vi "Extract K-Clock Phase Using Hilbert.vi"(7 "window":T1 items=["Rectangle"=0, "Hanning"=1, "Hamming"=2, "Blackman-Harris"=3, "Exact Blackman"=4, "Blackman"=5, "Flat Top"=6, "4 Term B-Harris "=7, "7 Term B-Harris"=8, "Low Sidelobe"=9, "Blackman Nuttall"=11, "Triangle"=30, "Bartlett-Hanning"=31, "Bohman"=32, "Parzen"=33, "Welch"=34, "Kaiser"=60, "Dolph-Chebyshev"=61, "Gaussian"=62], 11 "Input Data":dbl[](array[numeric]) format="%0.2f") -> (3 "Hilbert Unwrapped Phase":dbl[](array[numeric]))   [LabVIEW 2012]
uses:
  <vilib>/Analysis/4window.llb/windowTd.ctl
  <vilib>/Analysis/baseanly.llb/Mean (DBL).vi
  <vilib>/Analysis/0measdsp.llb/Scaled Time Domain Window (DBL).vi
  <vilib>/Analysis/NI_AALPro.lvlib
  <vilib>/Analysis/NI_AALBase.lvlib
panel:
  out "Hilbert Phase":dbl[](graph)
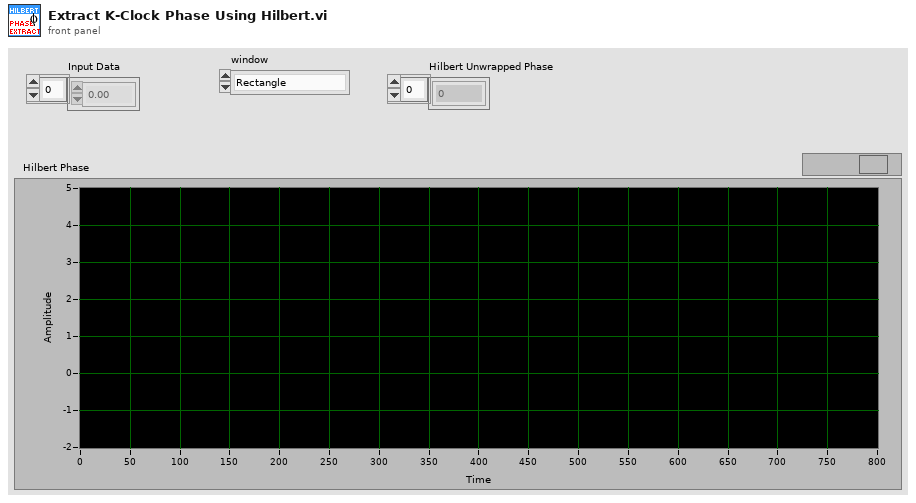
[diagram p1: front panel]
types:
  T1 = typedef "NI_AALPro.lvlib/windowTd.ctl" = u32
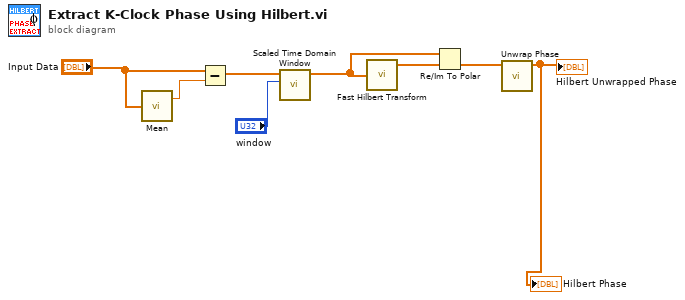
[diagram p0: block diagram]
diagram:
  n1 = call-poly <vilib>:"Mean.vi"("X"="Input Data") -> ("mean"=w8:dbl)  [unwired: 1 out]
  n2 = Subtract(x="Input Data", y=w8) -> (x-y=w4:dbl[])
  n3 = call-poly <vilib>:"Scaled Time Domain Window.vi"("window"="window", "X"=w4) -> ("Windowed X"=w3:dbl[])  [unwired: 7 in, 2 out]
  n4 = call <vilib>:"Fast Hilbert Transform.vi"("X"=w3) -> ("Hilbert{X}"=w7:dbl[])  [unwired: 1 out]
  n5 = Re/Im To Polar(2:w7, 3:w3) -> (0:w6:dbl[])  [unwired: 1 out]
  n6 = call <vilib>:"Unwrap Phase.vi"("Phase"=w6) -> ("Unwrapped Phase"=→"Hilbert Unwrapped Phase" →"Hilbert Phase":dbl[])  [unwired: 9 in, 1 out]
